vi "a.vi"   [LabVIEW 2018]
uses:
  Libraries/Thermal Chamber Response Simulator/Thermal Chamber Response Simulator.lvlib
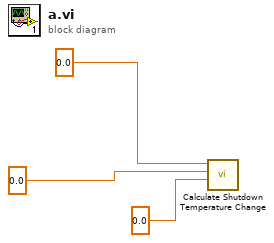
[diagram p0: block diagram]
diagram:
  n1 = call "Calculate Shutdown Temperature Change.vi"("Interval"=0.0, "Actual Temperature In"=0.0, "Required Temperature deg C"=0.0) -> ()  [unwired: 8 in, 1 out]
